vi "Reset Q0 error.vi"(8 "error in (no error)":errorcluster, 11 "Scope5761 in":refnum<class "Scope5782_six_channel.lvclass">) -> (0 "error out":errorcluster, 3 "Scope5761 out":refnum<class "Scope5782_six_channel.lvclass">)   [LabVIEW 2025, in "Scope5782_six_channel.lvclass"]
uses:
  Scope5782_six_channel.lvclass
  Scope5782_six_channel.lvclass/Scope5782_six_channel.ctl
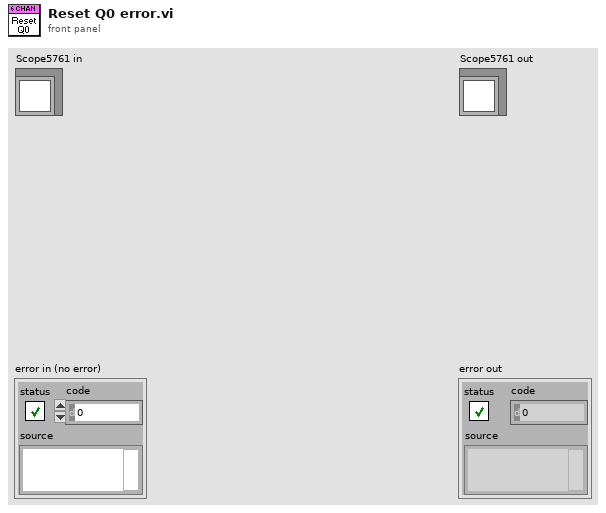
[diagram p1: front panel]
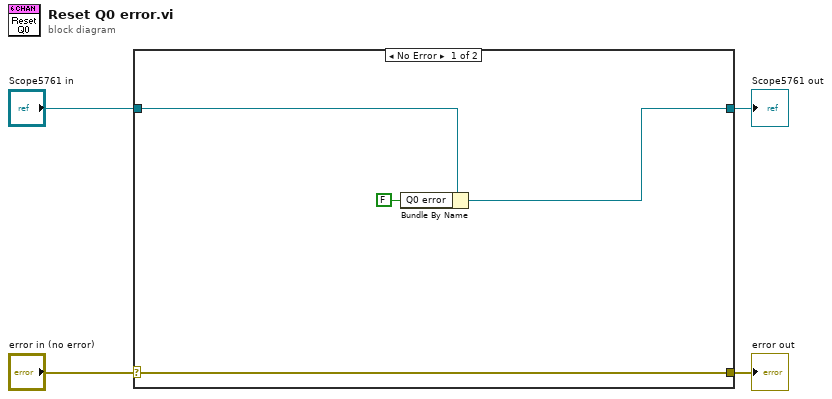
[diagram p0: block diagram]
diagram:
  n1 = case shown="No Error" "error in (no error)" {
    selector: "error in (no error)" -> [w8 w10]
    tunnel: [w8 w10] -> w3
    tunnel: [w5 w9] -> w1
    tunnel: "Scope5761 in" -> [w7 w9]
    frame No Error {
      n2 = Bundle By Name(cluster=w7, "Q0 error"=FALSE) -> (w5:refnum<class "Scope5782_six_channel.lvclass">)
    }
    frame Error {
    }
  }
  "error out" <- w3
  "Scope5761 out" <- w1
